vi "setFirstNumber.vi"(10 "firstNumber":dbl, 11 "View in":refnum<class "View.lvclass">) -> (3 "View out":refnum<class "View.lvclass">)   [LabVIEW 2016, in "View.lvclass"]
uses:
  View.lvclass
  View.lvclass/View.ctl
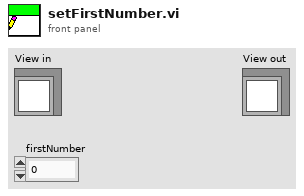
[diagram p1: front panel]
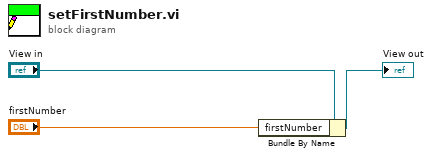
[diagram p0: block diagram]
diagram:
  n1 = Bundle By Name(cluster="View in", "firstNumber"="firstNumber") -> (→"View out":refnum<class "View.lvclass">)
